vi "Config-Display-Graphics-Line.vi"(5 "gradient":dbl format="%.4f", 6 "mode":i32(slide) max=3 scale=0.0..3.0, 7 "show line parameters":bool=TRUE, 8 "error in (no error)":errorcluster, 9 "state":bool=TRUE, 10 "active line":bool=TRUE, 11 "VISA session":refnum<visa-resource-name>) -> (0 "error out":errorcluster, 3 "VISA resource name out":refnum<visa-resource-name>)   [LabVIEW 2016, in "Agilent 415X Series.lvlib"]
doc: "This VI controls the lines which can be displayed on the GRAPHIC display.\n\nThis VI automatically switches the display mode to GRAPHIC."
uses:
  Agilent 415X Series.lvlib
panel:
  # "This VI selects GRAPHICS display mode automatically."
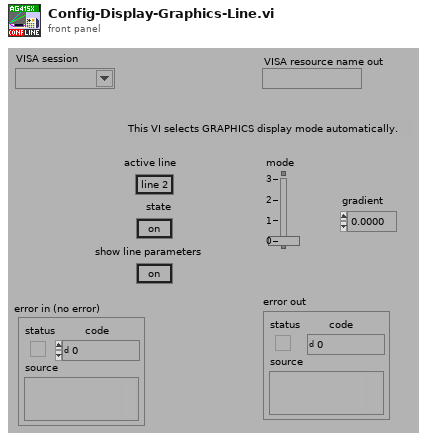
[diagram p1: front panel]
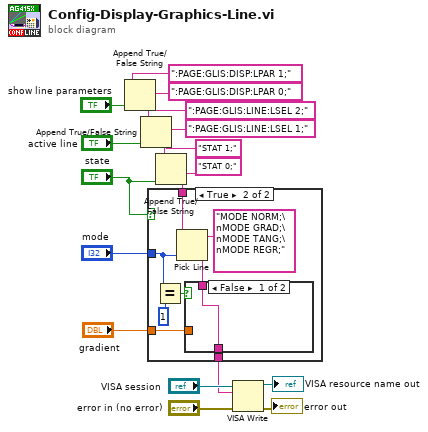
[diagram p0: block diagram]
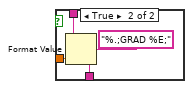
[diagram p3: hidden frame]
diagram:
  n1 = Append True/False String(1:"show line parameters", 2:":PAGE:GLIS:DISP:LPAR 0;", 3:":PAGE:GLIS:DISP:LPAR 1;") -> (0:w4:string)  [unwired: 1 in]
  n2 = Append True/False String(1:"active line", 2:":PAGE:GLIS:LINE:LSEL 1;", 3:":PAGE:GLIS:LINE:LSEL 2;", 4:w4) -> (0:w14:string)
  n3 = Append True/False String(1:"state", 2:"STAT 0;", 3:"STAT 1;", 4:w14) -> (0:w9:string)
  n4 = case shown="True" "state" {
    tunnel: w9 -> [w20 w28]
    tunnel: "mode" -> [_ w25]
    tunnel: "gradient" -> [_ w26]
    tunnel: [w20 w22] -> w2
    frame False {
      # "line state: off"
    }
    frame True {
      n5 = Equal?(x=w25, y=1) -> (x = y?=w23:bool)
      n6 = Pick Line(string ("")=w28, multi-line string="MODE NORM;\nMODE GRAD;\nMODE TANG;\nMODE REGR;", line index=w25) -> (output string=w27:string)
      n7 = case shown="False" w23 {
        tunnel: w27 -> [w29 w33]
        tunnel: w26 -> [_ w32]
        tunnel: [w29 w30] -> w22
        frame False {
        }
        frame True {
          n8 = Format Value(string ("")=w33, format string="%.;GRAD %E;", value (0)=w32) -> (output string=w30:string)
        }
      }
    }
  }
  n9 = VISA Write(VISA resource name="VISA session", write buffer=w2, error in (no error)="error in (no error)") -> (VISA resource name out=→"VISA resource name out":refnum<visa-resource-name>, error out=→"error out":errorcluster)  [unwired: 1 out]
